vi "TWM Client Cmd Define Multiplexer Paths.vi"(5 "timeout [ms]":i32=5000, 7 "end of packet key":string="TWM:command:EndOfPacket", 8 "error in":errorcluster, 10 "mux paths":T1[](array[typedef]), 11 "handle":i32) -> (0 "error out":errorcluster, 3 "handle out":i32)   [LabVIEW 2020, in "TWM Client.lvlib"]
doc: "This will define multiplexer paths. It is equivalent to manual definition of paths (channels) in multiplexer panel. It works only for generic multiplexers (some of them). Otherwise it do nothing."
uses:
  TWM Client.lvlib
  TWM Client Mux Path.ctl
  1D String.vi
  infolib.lvlib
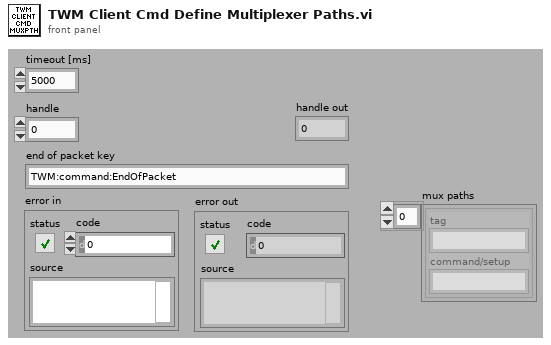
[diagram p1: front panel]
types:
  T1 = typedef "TWM Client.lvlib/TWM Client Mux Path.ctl" = cluster{"tag":string, "command/setup":string}
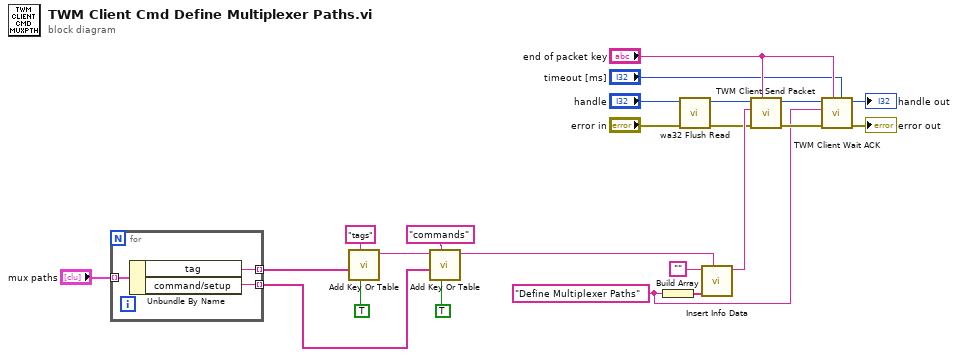
[diagram p0: block diagram]
diagram:
  w16 = "Define Multiplexer Paths" ("section name")
  n1 = for {
    tunnel: "mux paths" -> [w26] mode=indexing
    tunnel: [w25] -> w12 mode=indexing
    tunnel: [w24] -> w6 mode=indexing
    n2 = Unbundle By Name(w26) -> ("tag"=w25:string, "command/setup"=w24:string)
  }
  n3 = call-poly "Add Key Or Table.vi"("collumn vector (F)"=TRUE, "key description"="tags", "string"=w12) -> ("info data out"=w7:string)  [unwired: 7 in, 1 out]
  n4 = call-poly "Add Key Or Table.vi"("collumn vector (F)"=TRUE, "key description"="commands", "string"=w6, "info data"=w7) -> ("info data out"=w5:string)  [unwired: 6 in, 1 out]
  n5 = Build Array(w16) -> (w22:string[])
  n6 = call "wa32 Flush Read.vi"("error in"="error in", "handle"="handle") -> ("error out"=w3:errorcluster, "handle out"=w2:i32)  [unwired: 7 in, 1 out]
  n7 = call "Insert Info Data.vi"("info data to insert"=w5, "sections"=w22, "info data"="") -> ("info data out"=w23:string)  [unwired: 7 in, 1 out]
  n8 = call "TWM Client Send Packet.vi"("end of packet key"="end of packet key", "error in"=w3, "command string"=w23, "handle"=w2) -> ("error out"=w18:errorcluster, "handle out"=w15:i32)  [unwired: 6 in]
  n9 = call "TWM Client Wait ACK.vi"("timeout [ms] (3000)"="timeout [ms]", "key string"="end of packet key", "error in"=w18, "command header"=w16, "handle"=w15) -> ("error out"=→"error out":errorcluster, "handle out"=→"handle out":i32)  [unwired: 5 in]
